vi "Broadcast to Guardians.vi"(4 "Critical PCs also?":bool=TRUE, 5 "Message Priority":T1=enum."Normal", 6 "Only active ones?":bool=TRUE, 7 "Local also?":bool, 8 "error in (no error)":errorcluster, 9 "Data":variant, 10 "Message":string, 11 "Guardian in":refnum<class "Guardian.lvclass">) -> (0 "error out":errorcluster, 3 "Guardian out":refnum<class "Guardian.lvclass">)   [LabVIEW 2026, in "TALOS.lvlib" / "Guardian.lvlib" / "Guardian.lvclass"]
doc: "This VI sends a message to all the other Guardians, by writing it on Broadcast_Guardian SV."
uses:
  Guardian.lvclass
  C:/LabVIEW Code/TALOS/builds/Actor Framework PPL/Actor Framework.lvlibp/1abvi3w/vi.lib/ActorFramework/Actor/Actor.lvclass
  C:/LabVIEW Code/TALOS/talos/Ancestor/Ancestor/Ancestor.lvclass
  builds/Actor Framework PPL/Actor Framework.lvlibp/1abvi3w/vi.lib/ActorFramework/Message Enqueuer/Message Priority.ctl
  Guardian.lvclass/Guardian.ctl
  Ancestor/Ancestor/Ancestor.lvclass/Ancestor.ctl
  Guardian Messages/Message to Other Guardian Msg/Message to Other Guardian Msg.lvclass/Message to Other Guardian Msg.ctl
  Guardian Messages/TCP-SV Message Interpreter Msg/TCP-SV Message Interpreter Msg.lvclass/TCP-SV Message Interpreter Msg.ctl
  Support VIs/Generate Error.vi
  FGV/Error Memory/Get Error Description.vi
  Support VIs/Get PC name.vi
  Support VIs/Get Class Name.vi
  <vilib>/Utility/error.llb/Clear Errors.vi
  FGV/Error Memory/Error Memory Core.vi
  <vilib>/AdvancedString/Delimited String to 1D String Array.vi
  <vilib>/AdvancedString/Delimited String to 1D String Array (string).vi
  Support VIs/Circus Root Path.vi
  FGV/Error Memory/Error Crt Lvl checker.vi
  FGV/Error Memory/Error Memory Core.vi/40c8088d-b597-4017-91af-faa98e00292e.vi
  FGV/Error Memory/Error Memory Core.vi/d4a3ab98-063c-4e44-b43d-fbdcfe6c2be2.vi
  Support VIs/Global Constants.vi
  builds/Actor Framework PPL/Actor Framework.lvlibp/1abvi3w/vi.lib/ActorFramework/Message Enqueuer/Enqueue.vi
  Support VIs/Global Memory.vi
  <vilib>/Utility/LVClass/Get LV Class Name.vi
  Support VIs/Is in Packed Library.vi
  Support VIs/TALOS Root path.vi
  Support VIs/Read CSV worksheet.vi
  <vilib>/Utility/error.llb/General Error Handler.vi
  Support VIs/Error Log.vi
  Guardian Messages/Message to Other Guardian Msg/Message to Other Guardian Msg.lvclass
  Guardian Messages/TCP-SV Message Interpreter Msg/TCP-SV Message Interpreter Msg.lvclass
  Ancestor/Ancestor/Ancestor.lvclass
  <vilib>/Comparison/Equal/Equal Functor/Equal Functor.lvclass
  Classes/Guardian List/Guardian List.lvclass
  builds/Actor Framework PPL/Actor Framework.lvlibp/1abvi3w/vi.lib/ActorFramework/Actor/Actor.lvclass
  TALOS.lvlib
  builds/Actor Framework PPL/Actor Framework.lvlibp/1abvi3w/vi.lib/ActorFramework/Message Enqueuer/Message Enqueuer.lvclass
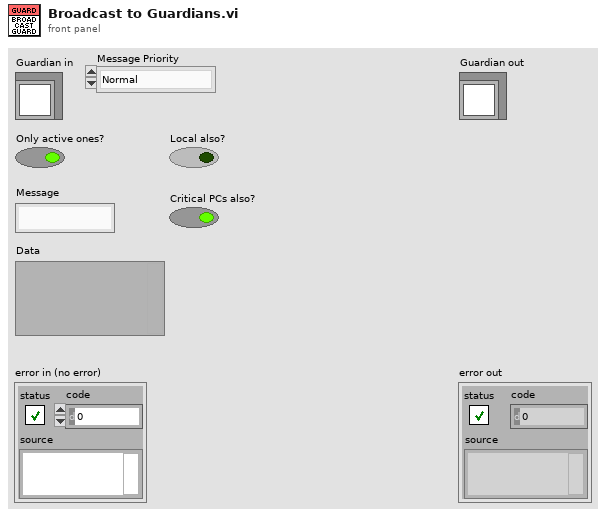
[diagram p1: front panel]
types:
  T1 = typedef "Actor Framework.lvlibp/Message Enqueuer.lvclass/Message Priority.ctl" = enum16{"Low", "Normal", "High"}
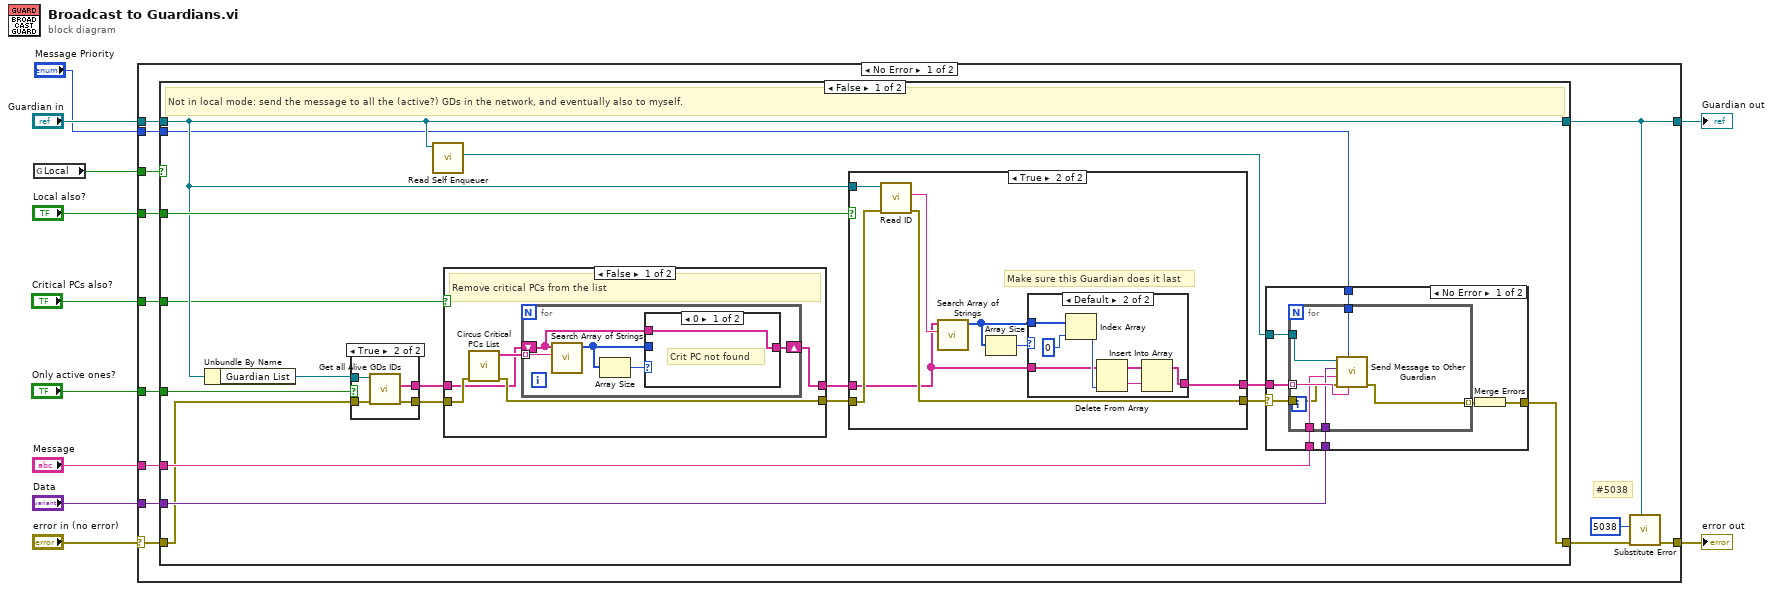
[diagram p0: block diagram]
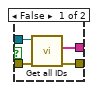
[diagram p2: hidden frame]
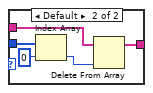
[diagram p3: hidden frame]
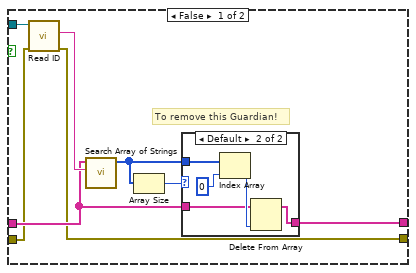
[diagram p5: hidden frame]
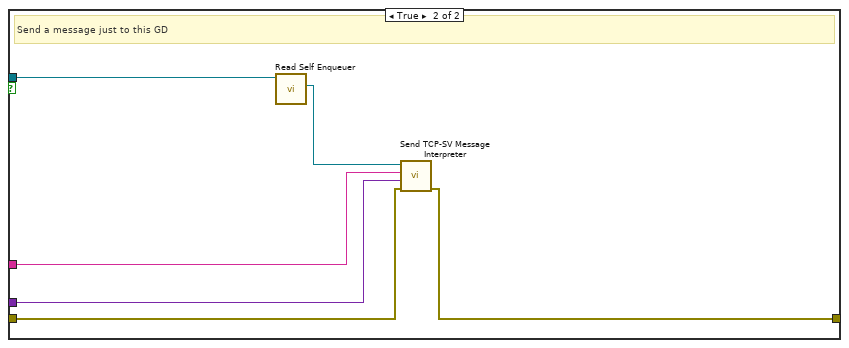
[diagram p10: hidden frame]
diagram:
  n1 = global read "Global Constants.vi" "Local"() -> (w3:bool)
  n2 = case shown="No Error" "error in (no error)" {
    selector: "error in (no error)" -> [w20 w128]
    tunnel: [w16 w128] -> w10
    tunnel: [w15 w127] -> w8
    tunnel: "Guardian in" -> [w22 w127]
    tunnel: "Message" -> [w24 _]
    tunnel: "Data" -> [w23 _]
    tunnel: "Only active ones?" -> [w21 _]
    tunnel: "Local also?" -> [w19 _]
    tunnel: w3 -> [w18 _]
    tunnel: "Critical PCs also?" -> [w13 _]
    tunnel: "Message Priority" -> [w12 _]
    frame No Error {
      # "#5038"
      n3 = case shown="False" w18 {
        tunnel: [w41 w117] -> w17
        tunnel: w24 -> [w40 w115]
        tunnel: w23 -> [w39 w114]
        tunnel: w22 -> [w32 w116]
        tunnel: w21 -> [w36 _]
        tunnel: w20 -> [w35 w118]
        tunnel: w19 -> [w34 w119]
        tunnel: [w32 w116] -> w15
        tunnel: w13 -> [w31 _]
        tunnel: w12 -> [w25 _]
        frame False {
          # "Not in local mode: send the message to all the (active?) GDs in the network, and eventually also to myself."
          n4 = Unbundle By Name(w32) -> ("Guardian List"=w26:refnum<class "Guardian List.lvclass">)
          n5 = case shown="True" w36 {
            tunnel: w26 -> [w45 w49]
            tunnel: [w43 w47] -> w30
            tunnel: w35 -> [w44 w48]
            tunnel: [w42 w46] -> w29
            frame False {
              n6 = call-dynamic "Get all IDs.vi"("error in (no error)"=w44, "Guardian List in"=w45) -> ("error out"=w42:errorcluster, "All IDs"=w43:string[])  [unwired: 7 in, 1 out]
            }
            frame True {
              n7 = call-dynamic "Get all Alive GDs IDs.vi"("error in (no error)"=w48, "Guardian List in"=w49) -> ("error out"=w46:errorcluster, "Alive GDs IDs"=w47:string[])  [unwired: 7 in, 1 out]
            }
          }
          n8 = call "Read Self Enqueuer.vi"("Actor"=w32) -> ("Self Enqueuer"=w38:refnum<class "Message Enqueuer.lvclass">)  [unwired: 10 in]
          n9 = case shown="False" w31 {
            tunnel: w30 -> [w50 w67]
            tunnel: w29 -> [w54 w66]
            tunnel: [w52 w67] -> w28
            tunnel: [w51 w66] -> w27
            frame False {
              # "Remove critical PCs from the list"
              n10 = call "Circus Critical PCs List.vi"("error in (no error)"=w54) -> ("error out"=w51:errorcluster, "Critical PC List out"=w53:string[])  [unwired: 9 in]
              n11 = for {
                tunnel: w53 -> [w59] mode=indexing
                shift-right: [w57] -> w52
                shift-left: w50 -> [w58]
                n12 = call "Search Array of Strings.vi"("search string"=w59, "Search array"=w58) -> ("indices"=w56:i32[])  [unwired: 8 in, 1 out]
                n13 = Array Size(array=w56) -> (size(s)=w55:i32)
                n14 = case shown="0" w55 {
                  tunnel: w56 -> [_ w64]
                  tunnel: w58 -> [w60 w62]
                  tunnel: [w60 w61] -> w57
                  frame 0 {
                    # "Crit PC not found"
                  }
                  frame Default {
                    n15 = Index Array(array=w64, index=0) -> (element=w63:i32)
                    n16 = Delete From Array(array=w62, index=w63) -> (array with subset deleted=w61:string[])  [unwired: 1 in, 1 out]
                  }
                }
              }
            }
            frame True {
              # "Sending to everything"
            }
          }
          n17 = case shown="True" w34 {
            tunnel: w32 -> [w75 w88]
            tunnel: [w73 w85] -> w37
            tunnel: w28 -> [w72 w84]
            tunnel: w27 -> [w71 w87]
            tunnel: [w70 w86] -> w33
            frame False {
              # "To remove this Guardian!"
              n18 = call "Read ID.vi"("error in (no error)"=w71, "Ancestor in"=w75) -> ("error out"=w70:errorcluster, "ID"=w74:string)  [unwired: 7 in, 1 out]
              n19 = call "Search Array of Strings.vi"("search string"=w74, "Search array"=w72) -> ("indices"=w69:i32[])  [unwired: 8 in, 1 out]
              n20 = Array Size(array=w69) -> (size(s)=w68:i32)
              n21 = case shown="Default" w68 {
                tunnel: [w76 w77] -> w73
                tunnel: w72 -> [w76 w79]
                tunnel: w69 -> [_ w78]
                frame 0 {
                  # "PC not found"
                }
                frame Default {
                  n22 = Index Array(array=w78, index=0) -> (element=w80:i32)
                  n23 = Delete From Array(array=w79, index=w80) -> (array with subset deleted=w77:string[])  [unwired: 1 in, 1 out]
                }
              }
            }
            frame True {
              # "Make sure this Guardian does it last"
              n24 = call "Read ID.vi"("error in (no error)"=w87, "Ancestor in"=w88) -> ("error out"=w86:errorcluster, "ID"=w89:string)  [unwired: 7 in, 1 out]
              n25 = call "Search Array of Strings.vi"("search string"=w89, "Search array"=w84) -> ("indices"=w82:i32[])  [unwired: 8 in, 1 out]
              n26 = Array Size(array=w82) -> (size(s)=w83:i32)
              n27 = case shown="Default" w83 {
                tunnel: [w90 w92] -> w85
                tunnel: w84 -> [w90 w95]
                tunnel: w82 -> [_ w94]
                frame 0 {
                  # "PC not found"
                }
                frame Default {
                  n28 = Index Array(array=w94, index=0) -> (element=w96:i32)
                  n29 = Delete From Array(array=w95, index=w96) -> (deleted portion=w91:string, array with subset deleted=w93:string[])  [unwired: 1 in]
                  n30 = Insert Into Array(array=w93, new element=w91) -> (w92:string[])  [unwired: 1 in]
                }
              }
            }
          }
          n31 = case shown="No Error" w33 {
            selector: w33 -> [w99 w113]
            tunnel: [w105 w113] -> w41
            tunnel: w40 -> [w103 _]
            tunnel: w39 -> [w102 _]
            tunnel: w38 -> [w101 _]
            tunnel: w37 -> [w100 _]
            tunnel: w25 -> [w98 _]
            frame No Error {
              n32 = for {
                tunnel: [w108] -> w104 mode=indexing
                tunnel: w100 -> [w111] mode=indexing
                tunnel: w103 -> [w109]
                tunnel: w102 -> [w110]
                tunnel: w101 -> [w112]
                tunnel: w99 -> [w107]
                tunnel: w98 -> [w106]
                n33 = call "Send Message to Other Guardian.vi"("Guardian ID"=w111, "Message Priority (Normal)"=w106, "error in (no error)"=w107, "Message"=w109, "Data"=w110, "Message Enqueuer"=w112) -> ("error out"=w108:errorcluster)  [unwired: 4 in, 1 out]
              }
              n34 = Merge Errors(w104) -> (w105:errorcluster)
            }
            frame Error {
            }
          }
        }
        frame True {
          # "Local mode!"
          n35 = case shown="False" w119 {
            tunnel: w118 -> [w120 w122]
            tunnel: [w120 w121] -> w117
            tunnel: w116 -> [_ w126]
            tunnel: w115 -> [_ w124]
            tunnel: w114 -> [_ w123]
            frame False {
              # "Do nothing then!"
            }
            frame True {
              # "Send a message just to this GD"
              n36 = call "Read Self Enqueuer.vi"("Actor"=w126) -> ("Self Enqueuer"=w125:refnum<class "Message Enqueuer.lvclass">)  [unwired: 10 in]
              n37 = call "Send TCP-SV Message Interpreter.vi"("error in (no error)"=w122, "Data"=w123, "Message"=w124, "Message Enqueuer"=w125) -> ("error out"=w121:errorcluster)  [unwired: 6 in, 1 out]
            }
          }
        }
      }
      n38 = call "Substitute Error.vi"("LabVIEW Object"=w15, "error in (no error)"=w17, "Error Code"=5038) -> ("error out"=w16:errorcluster)  [unwired: 8 in]
    }
    frame Error {
    }
  }
  "error out" <- w10
  "Guardian out" <- w8
